vi "Prober_ChuckUpDown.vi"(8 "error in (no error)":errorcluster, 10 "Direction":enum16{"up", "down"}(ring), 11 "ProbeStationControl in":refnum<class "ProbeStationControl.lvclass">) -> (0 "error out":errorcluster, 2 "Chuck at CONTACT?":bool=TRUE, 3 "ProbeStationControl out":refnum<class "ProbeStationControl.lvclass">)   [LabVIEW 2013, in "ProbeStationControl.lvclass"]
uses:
  ProbeStationControl.lvclass
  ProbeStationControl.lvclass/ProbeStationControl.ctl
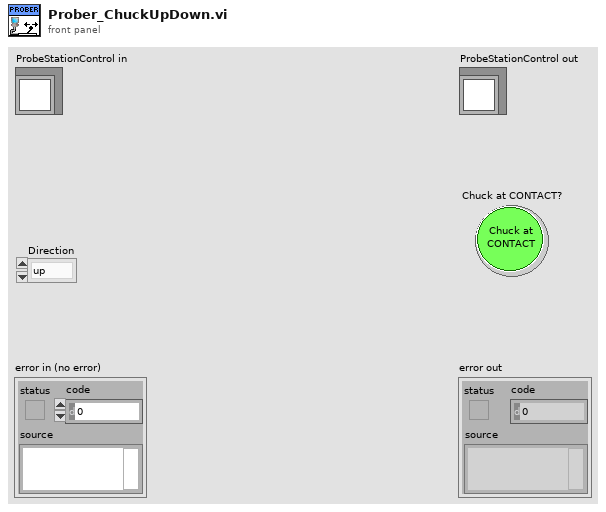
[diagram p1: front panel]
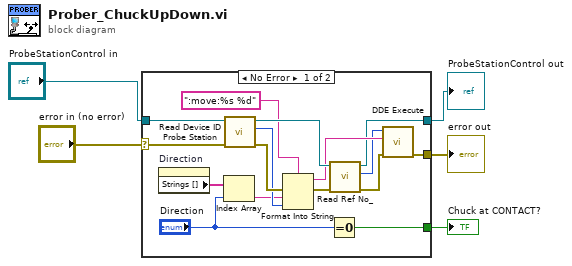
[diagram p0: block diagram]
diagram:
  n1 = case shown="No Error" "error in (no error)" {
    selector: "error in (no error)" -> [w14 w23]
    tunnel: [w10 w23] -> w4
    tunnel: "ProbeStationControl in" -> [w9 w22]
    tunnel: [w7 _] -> w3
    tunnel: [w6 w22] -> w1
    frame No Error {
      n2 = property on="Direction" class="Enum (strict)"() -> ("Strings []"=w21:string[])  [unwired: 2 in, 2 out]
      n3 = Index Array(array=w21, index="Direction") -> (element=w15:string)
      n4 = call "Read Device ID Probe Station.vi"("error in (no error)"=w14, "ProbeStationControl in"=w9) -> ("error out"=w18:errorcluster, "Device ID Probe Station"=w16:u32, "ProbeStationControl out"=w20:refnum<class "ProbeStationControl.lvclass">)  [unwired: 7 in]
      n5 = Format Into String(format string=":move:%s %d", error in=w18, w15, w16) -> (resulting string=w13:string, error out=w19:errorcluster)  [unwired: 1 in]
      n6 = Equal To 0?(x="Direction") -> (x = 0?=w7:bool)
      n7 = call "Read Ref No_.vi"("error in (no error)"=w19, "ProbeStationControl in"=w20) -> ("error out"=w11:errorcluster, "Ref No."=w12:i32, "ProbeStationControl out"=w6:refnum<class "ProbeStationControl.lvclass">)  [unwired: 7 in]
      n8 = call <vilib>:"DDE Execute.vi"("error in (no error)"=w11, "command"=w13, "conversation refnum in"=w12) -> ("error out"=w10:errorcluster)  [unwired: 5 in, 1 out]
    }
    frame Error {
    }
  }
  "error out" <- w4
  "Chuck at CONTACT?" <- w3
  "ProbeStationControl out" <- w1
